vi "Scan For Loop.vi"(0 "UI SA en entrée":refnum<class "UI SmarAct.lvclass">, 1 "itération":i32, 5 "Inc:(um)":dbl, 7 "PosX.Curs-1":dbl, 9 "Début (um)":i32, 11 "error in (no error)":errorcluster caption="entrée d'erreur (pas d'erreur)", 12 "PosX.Curs-0":dbl) -> (3 "Nbr de Scans":i32, 4 "UI SA en sortie":refnum<class "UI SmarAct.lvclass">, 6 "Aire":dbl, 14 "Spectrogramme One Acq":dbl[][](array[numeric]), 15 "error out":errorcluster caption="sortie d'erreur")   [LabVIEW 2024, in "UI SmarAct.lvclass"]
uses:
  UI SmarAct.lvclass
  UI SmarAct.lvclass/UI SmarAct.ctl
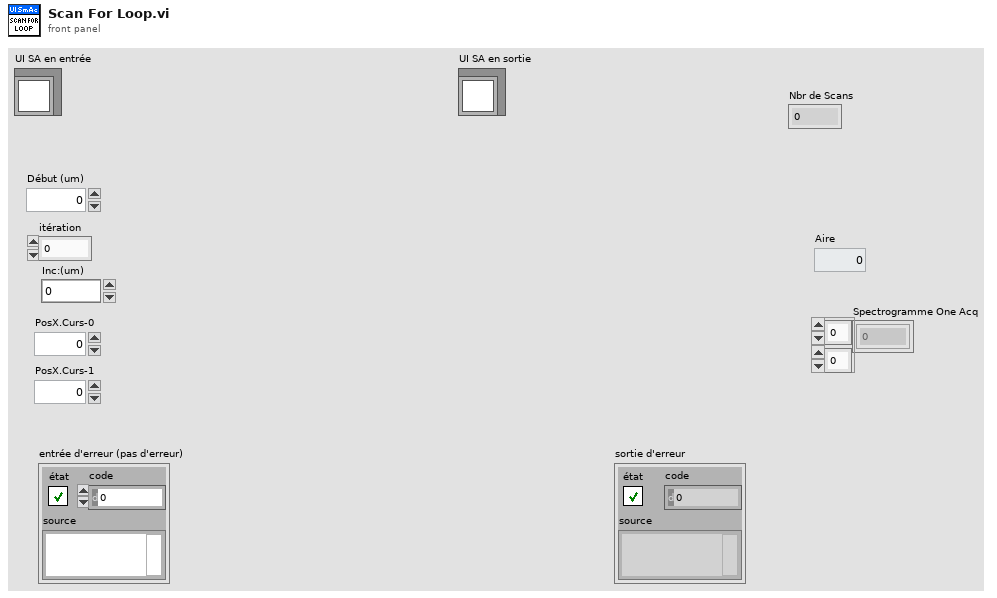
[diagram p1: front panel]
types:
  T1 = typedef "Spectro Acquisition.lvclass/rwr_One Acquisition Reply.ctl" = cluster{"Spectre-BKG":dbl[], "Nbr de Scans":i32, "Spectrogramme One Acq":dbl[][]}
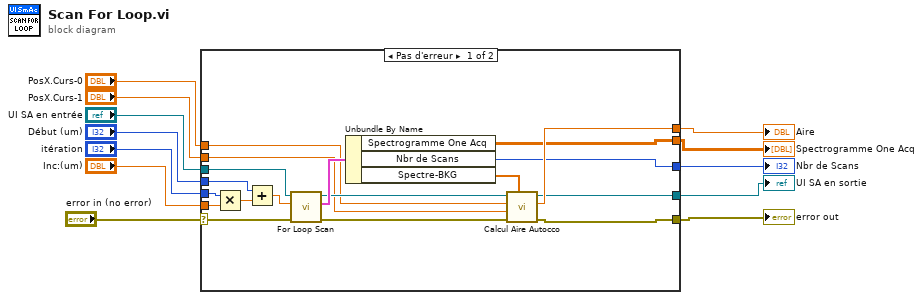
[diagram p0: block diagram]
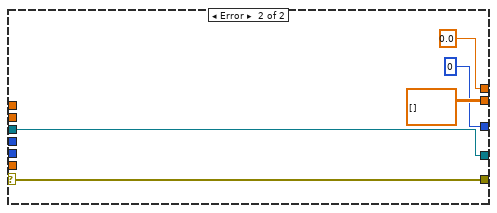
[diagram p2: hidden frame]
diagram:
  n1 = case shown="Pas d'erreur" "error in (no error)" {
    selector: "error in (no error)" -> [w18 w35]
    tunnel: [w17 w35] -> w11
    tunnel: [w13 w34] -> w9
    tunnel: "UI SA en entrée" -> [w14 w34]
    tunnel: "itération" -> [w24 _]
    tunnel: "Inc:(um)" -> [w23 _]
    tunnel: [w22 0.0 ("Aire Autocco")] -> w6
    tunnel: "PosX.Curs-0" -> [w21 _]
    tunnel: "PosX.Curs-1" -> [w20 _]
    tunnel: "Début (um)" -> [w19 _]
    tunnel: [w16 dbl[][] []] -> w2
    tunnel: [w15 0 ("Nbr de Scans")] -> w1
    frame No Error {
      n2 = Multiply(x=w24, y=w23) -> (x*y=w29:dbl)
      n3 = Add(x=w19, y=w29) -> (x+y=w28:dbl)
      n4 = call "For Loop Scan.vi"("error in (no error)"=w18, "Pas abs(um)"=w28, "UI SA en entrée"=w14) -> ("error out"=w27:errorcluster, "Reply Data out"=w30:T1, "UI SA en sortie"=w25:refnum<class "UI SmarAct.lvclass">)  [unwired: 6 in]
      n5 = Unbundle By Name(w30) -> ("Spectrogramme One Acq"=w16:dbl[][], "Nbr de Scans"=w15:i32, "Spectre-BKG"=w26:dbl[])
      n6 = call "Calcul Aire Autocco.vi"("Spectre-BKG"=w26, "error in (no error)"=w27, "PosX.Curs-1"=w20, "PosX.Curs-0"=w21, "UI SA en entrée"=w25) -> ("error out"=w17:errorcluster, "Aire Autocco"=w22:dbl, "UI SA en sortie"=w13:refnum<class "UI SmarAct.lvclass">)  [unwired: 4 in]
    }
    frame Error {
    }
  }
  "error out" <- w11
  "UI SA en sortie" <- w9
  "Aire" <- w6
  "Spectrogramme One Acq" <- w2
  "Nbr de Scans" <- w1
